vi "Results_CSV_Processing.vi"(8 "error in (no error)":errorcluster, 9 "Results":T1[](array[typedef]), 10 "Parameters":cluster{"Name":string, "Value":string}[](array[cluster]), 11 "file path (dialog if empty)":path) -> (0 "error out":errorcluster)   [LabVIEW 2020]
uses:
  XML Handler/Controls/Result Cluster.ctl
  <vilib>/Utility/file.llb/Write Delimited Spreadsheet (string).vi
  XML Handler/XML Handler.lvclass
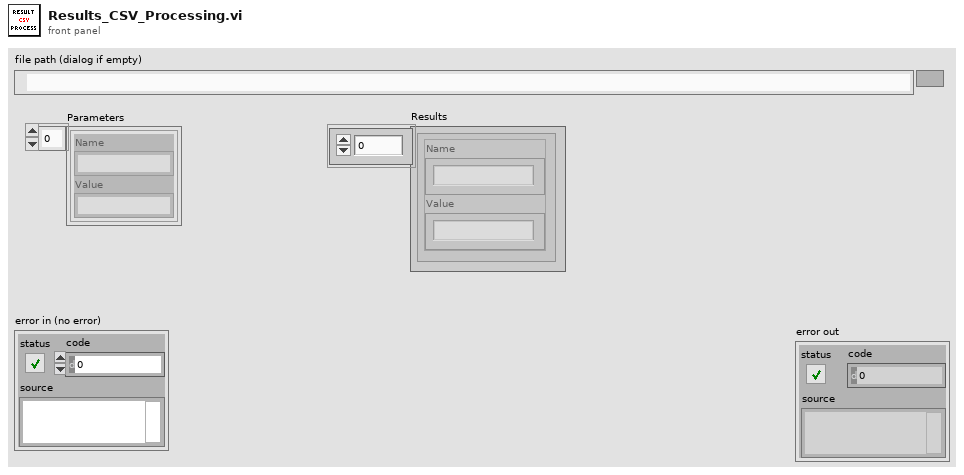
[diagram p1: front panel]
types:
  T1 = typedef "XML Handler.lvclass/Result Cluster.ctl" = cluster{"Name":string, "Value":string}
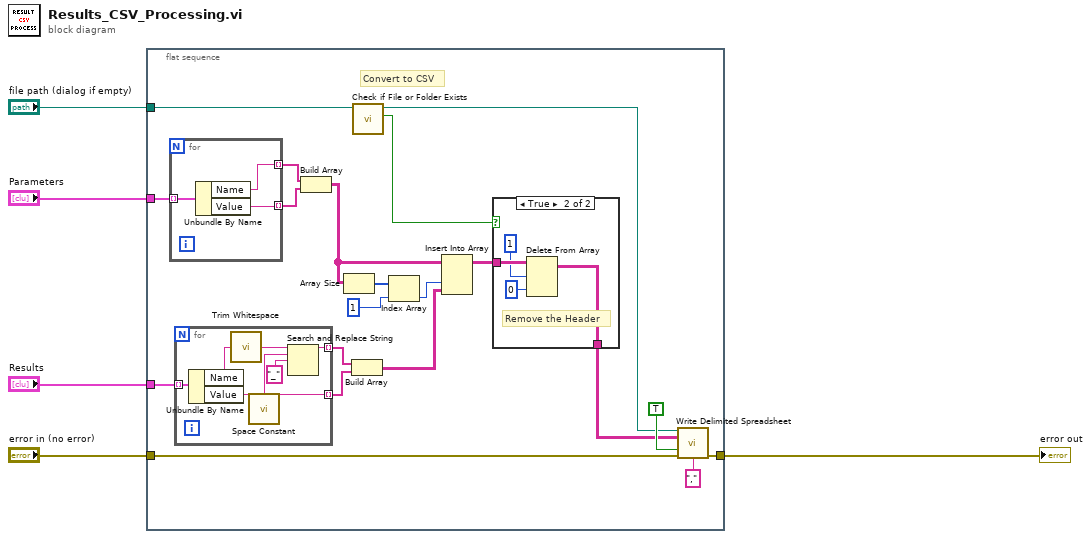
[diagram p0: block diagram]
diagram:
  n1 = flat-sequence {
    tunnel: "Results" -> [w25]
    tunnel: "file path (dialog if empty)" -> [w11]
    tunnel: "error in (no error)" -> [w6]
    tunnel: [w21] -> w2
    tunnel: "Parameters" -> [w20]
    frame #0 {
      # "Convert to CSV"
      n2 = for {
        tunnel: w20 -> [w33] mode=indexing
        tunnel: [w32] -> w19 mode=indexing
        tunnel: [w31] -> w18 mode=indexing
        n3 = Unbundle By Name(w33) -> ("Name"=w32:string, "Value"=w31:string)
      }
      n4 = for {
        tunnel: w25 -> [w40] mode=indexing
        tunnel: [w36] -> w24 mode=indexing
        tunnel: [w39] -> w23 mode=indexing
        n5 = Unbundle By Name(w40) -> ("Name"=w35:string, "Value"=w39:string)
        n6 = call <vilib>:"Trim Whitespace.vi"("string"=w35) -> ("trimmed string"=w34:string)  [unwired: 1 in]
        n7 = call <vilib>:"Space Constant.vi"() -> ("String"=w38:string)
        n8 = Search and Replace String(input string=w34, search string=w38, replace string="_" ("input string")) -> (result string=w36:string)  [unwired: 5 in, 3 out]
      }
      n9 = Build Array(w19, w18) -> (w16:string[][])
      n10 = Array Size(array=w16) -> (size(s)=w15:i32[])
      n11 = Build Array(w24, w23) -> (w17:string[][])
      n12 = call <vilib>:"Check if File or Folder Exists.vi"("path"=w11) -> ("file or folder exists?"=w9:bool, "dup path"=w7:path)  [unwired: 8 in, 1 out]
      n13 = Index Array(array=w15, index=1) -> (element=w13:i32)
      n14 = Insert Into Array(array=w16, index (col)=w13, new element=w17) -> (w10:string[][])  [unwired: 1 in]
      n15 = case shown="True" w9 {
        tunnel: w10 -> [w26 w30]
        tunnel: [w26 w27] -> w8
        frame False {
        }
        frame True {
          # "Remove the Header"
          n16 = Delete From Array(array=w30, length=1, index (row)=0) -> (array with subset deleted=w27:string[][])  [unwired: 1 in, 1 out]
        }
      }
      n17 = call-poly <vilib>:"Write Delimited Spreadsheet.vi"("file path (dialog if empty)"=w7, "2D data"=w8, "append to file? (new file:F)"=TRUE, "error in (no error)"=w6, "delimiter (\\t)"="," ("delimiter (\\t)")) -> ("error out"=w21:errorcluster)  [unwired: 9 in, 1 out]
    }
  }
  "error out" <- w2
